vi "StopMeas.vi"(8 "error in (no error)":errorcluster, 11 "NHRDCPower in":refnum<class "NHRDCPower.lvclass">) -> (0 "error out":errorcluster, 3 "NHRDCPower out":refnum<class "NHRDCPower.lvclass">)   [LabVIEW 2018, in "AcPwrPlugins.lvlib" / "NHRDCPower.lvclass"]
doc: "This VI stops the measurements."
uses:
  NHRDCPower.lvclass
  <instrlib>/NHRDCPowerModule/NHRDCPowerModule/NHRDCPowerModule.lvlib
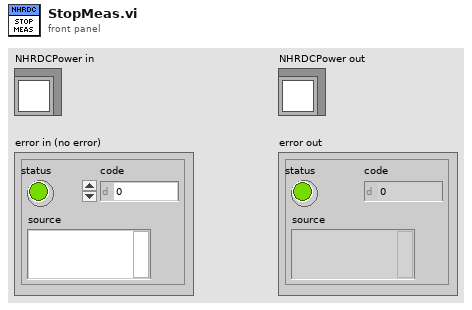
[diagram p1: front panel]
types:
  T1 = typedef "AcPwrPlugins.lvlib/NHRDCPower.lvclass/Measurements.ctl" = cluster{"Handle":string, "Name":string, "Enabled":bool, "Measurement Value":sgl, "btnMeasFetch":bool, "Measurement Type":i32, "Fetch Method":i32, "Fetch Time (s)":sgl}[]
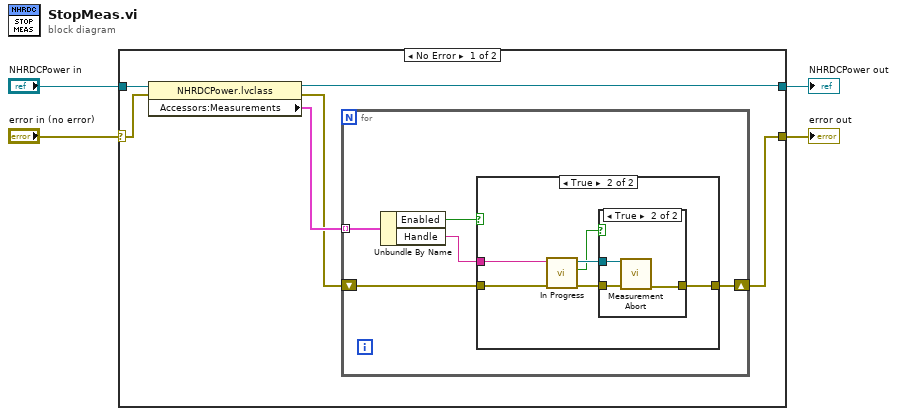
[diagram p0: block diagram]
diagram:
  n1 = case shown="No Error" "error in (no error)" {
    selector: "error in (no error)" -> [w9 w27]
    tunnel: [w5 w27] -> w1
    tunnel: [w6 w28] -> w2
    tunnel: "NHRDCPower in" -> [w10 w28]
    frame No Error {
      n2 = property class="NHRDCPower.lvclass"(reference=w10, error in=w9) -> (reference out=w6:refnum<class "NHRDCPower.lvclass">, error out=w7:errorcluster, "Accessors:Measurements"=w8:T1)
      n3 = for {
        tunnel: w8 -> [w15] mode=indexing
        shift-right: [w13] -> w5
        shift-left: w7 -> [w14]
        n4 = Unbundle By Name(w15) -> ("Enabled"=w12:bool, "Handle"=w11:string)
        n5 = case shown="True" w12 {
          tunnel: w14 -> [w16 w21]
          tunnel: [w16 w22] -> w13
          tunnel: w11 -> [_ w18]
          frame False {
          }
          frame True {
            n6 = call <instrlib>:"In Progress.vi"("error in (no error)"=w21, "instrument handle"=w18) -> ("error out"=w20:errorcluster, "in progress"=w17:bool, "instrument handle out"=w19:refnum<visa-resource-name>)  [unwired: 7 in]
            n7 = case shown="True" w17 {
              tunnel: w20 -> [w23 w26]
              tunnel: [w23 w24] -> w22
              tunnel: w19 -> [_ w25]
              frame False {
              }
              frame True {
                n8 = call <instrlib>:"Measurement Abort.vi"("error in (no error)"=w26, "instrument handle"=w25) -> ("error out"=w24:errorcluster)  [unwired: 8 in, 1 out]
              }
            }
          }
        }
      }
    }
    frame Error {
    }
  }
  "error out" <- w1
  "NHRDCPower out" <- w2
